vi "Pose2d_New.vi"(9 "Heading":dbl, 10 "Y":dbl, 11 "X":dbl) -> (3 "out POSe":T1 {"ROTATION"."SIN" format="%13.4f"; "ROTATION"."COS" format="%13.4f"; "ROTATION"."VALUE" format="%13.4f"; "TRANSLATION"."Y" format="%14.3f"; "TRANSLATION"."X" format="%14.3f"})   [LabVIEW 2019, in "Trajectory_Library.lvlib"]
doc: "Convenience constructors that takes in x and y values directly instead of having to construct a Translation2d.\n\nParameters:\n - X- The x component of the translational component of the pose.\n - Y - The y component of the translational component of the pose.\n - Rotation (Heading) - The rotational component of the pose.\n\nReturns:\n - OUT POSE - Output POSE"
uses:
  Trajectory_Library.lvlib
  TypeDef/TRANSLATION2D.ctl
  TypeDef/ROTATION2D.ctl
  TypeDef/POSE2D.ctl
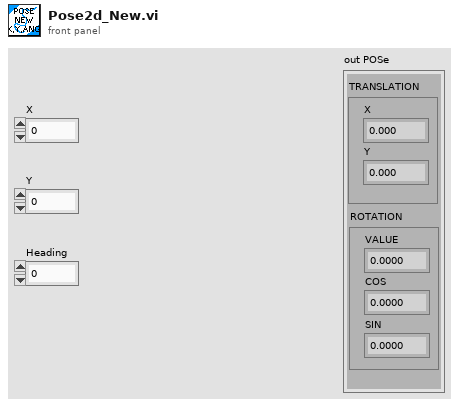
[diagram p1: front panel]
types:
  T1 = typedef "Trajectory_Library.lvlib/POSE2D.ctl" = cluster{"TRANSLATION":T2, "ROTATION":T3}
  T2 = typedef "Trajectory_Library.lvlib/TRANSLATION2D.ctl" = cluster{"X":dbl, "Y":dbl}
  T3 = typedef "Trajectory_Library.lvlib/ROTATION2D.ctl" = cluster{"VALUE":dbl, "COS":dbl, "SIN":dbl}
  T4 = typedef "WPILib_Math.lvlib/TRANSLATION2D.ctl" = cluster{"X":dbl, "Y":dbl}
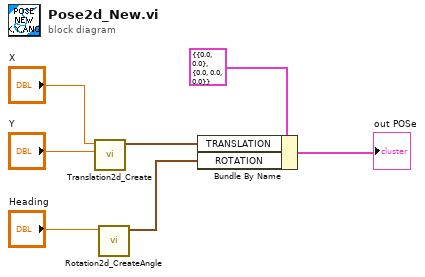
[diagram p0: block diagram]
diagram:
  n1 = call "Translation2d_Create.vi"("Y"="Y", "X"="X") -> ("TRANSLATION"=w3:T4)  [unwired: 9 in]
  n2 = call "Rotation2d_CreateAngle.vi"("Angle"="Heading") -> ("ROTATION"=w4:T3)  [unwired: 10 in]
  n3 = Bundle By Name(cluster=T1 {"TRANSLATION"={"X"=0.0, "Y"=0.0}, "ROTATION"={"VALUE"=0.0, "COS"=0.0, "SIN"=0.0}} ("sumPOSE"), "TRANSLATION"=w3, "ROTATION"=w4) -> (→"out POSe":T1)
